vi "CTRE_PigeonIMU_SetAccumZAngle.vi"(8 "error in (no error)":errorcluster, 10 "Angle (Deg)":dbl, 11 "PigeonIMUDevRef":T1={"DeviceStatus"={"status"=FALSE, "code"=0, "source"=""}, "Device Number"=0, "Type"=352321536, "Device ID"=0} {"Type" items=["CAN"=352321536, "TalonSRX"=33554432]}) -> (0 "error out":errorcluster, 3 "PigeonIMUDevRef":T1={"DeviceStatus"={"status"=FALSE, "code"=0, "source"=""}, "Device Number"=0, "Type"=352321536, "Device ID"=0} {"Type" items=["CAN"=352321536, "TalonSRX"=33554432]})   [LabVIEW 2016]
uses:
  <vilib>/Rock Robotics/WPI/ThirdParty/Sensors/Pigeon IMU/CTRE_PigeonIMU_DeviceRef.ctl
  <vilib>/Rock Robotics/WPI/ThirdParty/Sensors/Pigeon IMU/CTRE_PigeonIMU_ConnectionType.ctl
  <vilib>/Rock Robotics/WPI/ThirdParty/Sensors/Pigeon IMU/CTRE_PigeonIMU_TareType.ctl
  <vilib>/Rock Robotics/WPI/ThirdParty/Sensors/Pigeon IMU/CTRE_PigeonIMU_Params.ctl
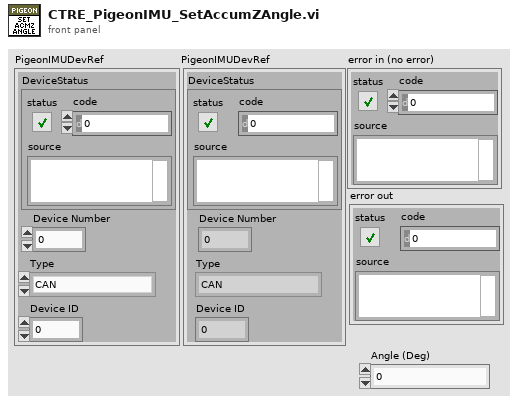
[diagram p1: front panel]
types:
  T1 = typedef "CTRE_PigeonIMU_DeviceRef.ctl" = cluster{"DeviceStatus":errorcluster, "Device Number":u8, "Type":T2, "Device ID":u32}
  T2 = typedef "CTRE_PigeonIMU_ConnectionType.ctl" = u32
  T3 = typedef "CTRE_PigeonIMU_Params.ctl" = u8
  T4 = typedef "CTRE_PigeonIMU_TareType.ctl" = u8
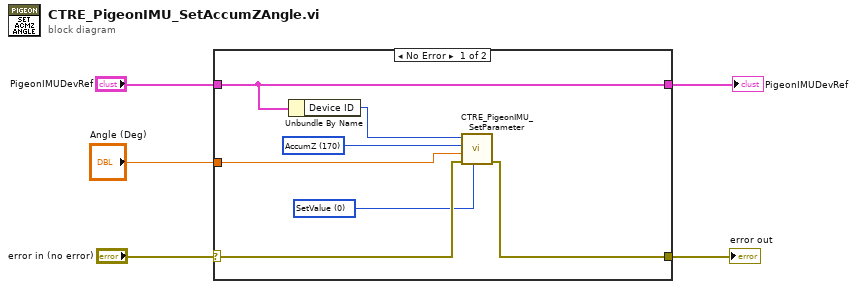
[diagram p0: block diagram]
diagram:
  n1 = case shown="No Error" "error in (no error)" {
    selector: "error in (no error)" -> [w9 w13]
    tunnel: [w8 w13] -> w4
    tunnel: [w12 w14] -> w2
    tunnel: "PigeonIMUDevRef" -> [w12 w14]
    tunnel: "Angle (Deg)" -> [w10 _]
    frame No Error {
      w6 = T3 170 items=["YawOffset"=160, "CompassOffset"=161, "BetaGain"=162, "Reserved163"=163, "GyroNoMotionCal"=164, "EnterCalibration"=165, "FusedHeadingOffset"=166, "StatusFrameRate"=169, "AccumZ"=170, "TempCompDisable"=171] ("Parameter")
      w7 = T4 0 items=["SetValue"=0, "AddOffset"=1, "MatchCompass"=2, "SetOffset"=255] ("TareType")
      n2 = Unbundle By Name(w12) -> ("Device ID"=w11:u32)
      n3 = call <vilib>:"CTRE_PigeonIMU_SetParameter.vi"("TareType"=w7, "error in (no error)"=w9, "Value"=w10, "Parameter"=w6, "Device ID (0)"=w11) -> ("error out"=w8:errorcluster)  [unwired: 5 in, 1 out]
    }
    frame Error {
    }
  }
  "PigeonIMUDevRef" <- w2
  "error out" <- w4
